vi "signal_generation_1.vi"() -> ()   [LabVIEW 2016]
uses:
  controls/State.ctl
  <vilib>/Utility/error.llb/DialogType.ctl
  <vilib>/DAQmx/write.llb/DAQmx Write (Analog Wfm 1Chan NSamp).vi
  <vilib>/DAQmx/write.llb/DAQmx Write (Analog DBL 1Chan 1Samp).vi
  <vilib>/DAQmx/read.llb/DAQmx Read (Analog 1D Wfm NChan NSamp).vi
  <vilib>/DAQmx/create/channels.llb/DAQmx Create Channel (AO-Voltage-Basic).vi
  <vilib>/DAQmx/create/channels.llb/DAQmx Create Channel (AI-Voltage-Basic).vi
  <vilib>/DAQmx/configure/timing.llb/DAQmx Timing (Sample Clock).vi
  <vilib>/DAQmx/miscellaneous.llb/DAQmx Fill In Error Info.vi
  <resource>/objmgr/daqmx.rc
  <vilib>/measure/NI_MABase.lvlib
panel:
  out "Waveform Graph 2":waveform(dbl)[](graph)=[{"t0"=timestamp(3594732894.3389087 s since 1904-01-01), "dt"=0.001, "Y"=array[1000 elements], "attributes"=variant("NI_ChannelName"=variant(string "DAQ_6363/ai0"), "NI_UnitDescription"=variant(string "Volts"))}]
  in  "DAQ channel 3 In":tag="DAQ_6363/ai0"
  out "error out":errorcluster
  in  "Number of Samples":i32=1000
  in  "Samples per Period":dbl=100.0
  in  "DAQ channel 2 In":tag="DAQ_6363/ao1"
  in  "DAQ channel 1 In":tag="DAQ_6363/ao0"
  in  "Error In (no error)":errorcluster
  in  "Exit Button":bool
  out "Status":string="Off"
  in  "TMA Voltage On/Off":bool
  out "Waveform Graph":waveform(dbl)(graph)={"t0"=timestamp(0 s since 1904-01-01), "dt"=0.001, "Y"=array[1000 elements]}
  in  "TMA Voltage":dbl=2.0 min=-10.0 max=10.0
  in  "Period (ms)":dbl=100.0 min=0.01
  in  "Amplitude (V)":dbl=2.0 min=0.0 max=30.0
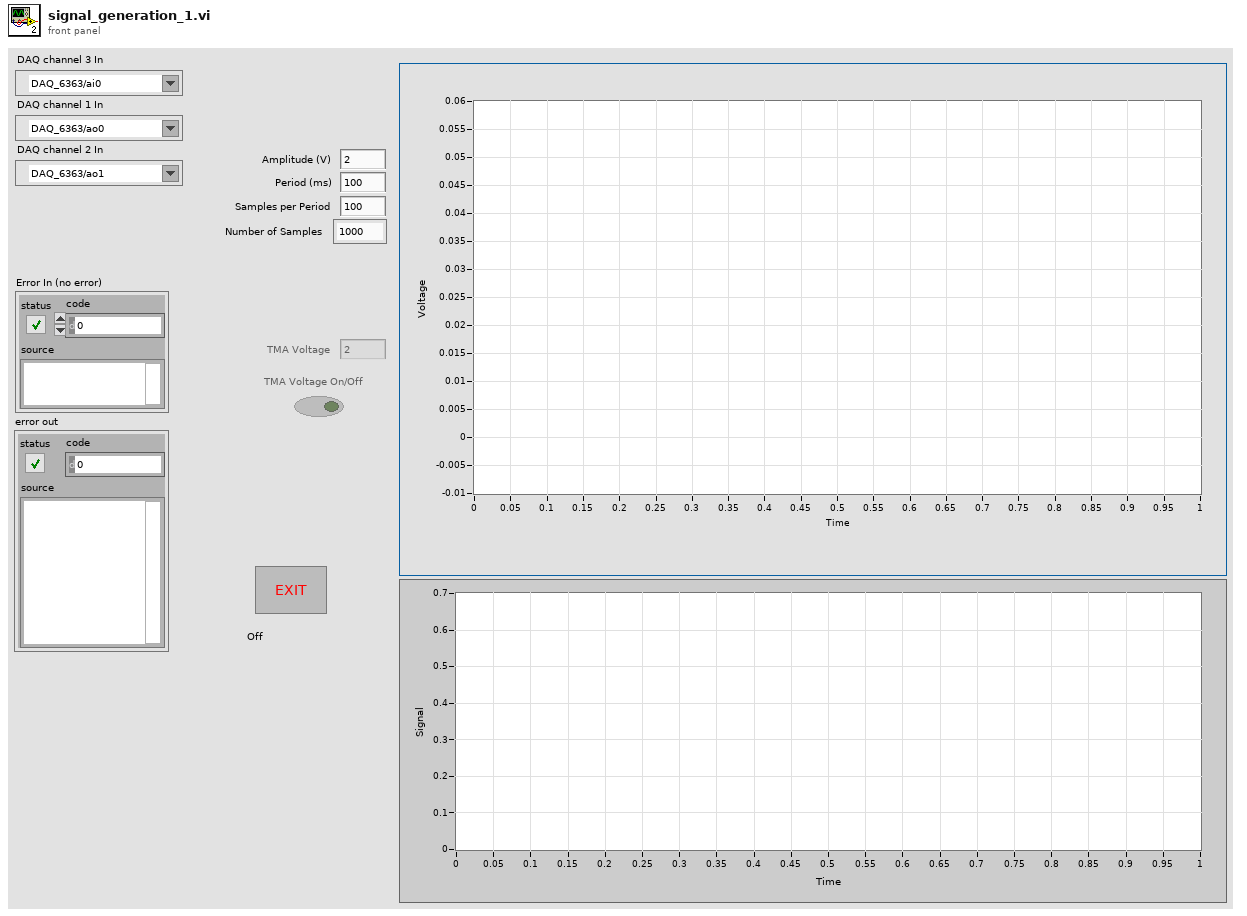
[diagram p1: front panel]
types:
  T1 = typedef "State.ctl" = enum16{"Init", "Idle", "Shutdown"}
  T2 = enum16{"Sine Wave", "Triangle Wave", "Square Wave", "Sawtooth Wave"}
  T3 = typedef "DialogType.ctl" = u16
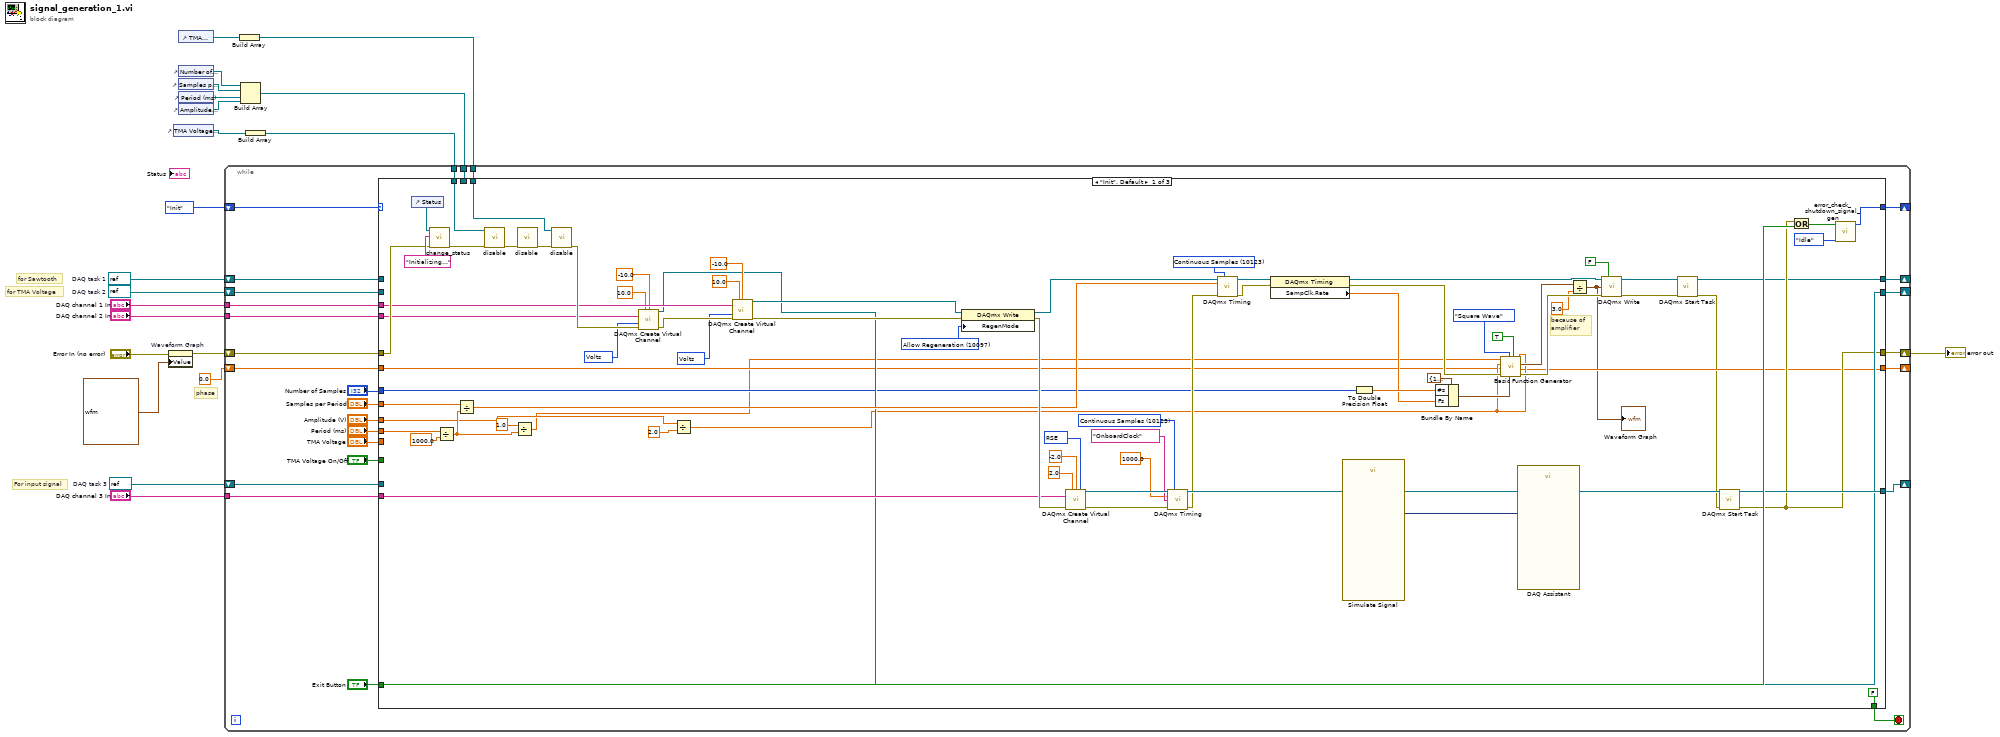
[diagram p0: block diagram]
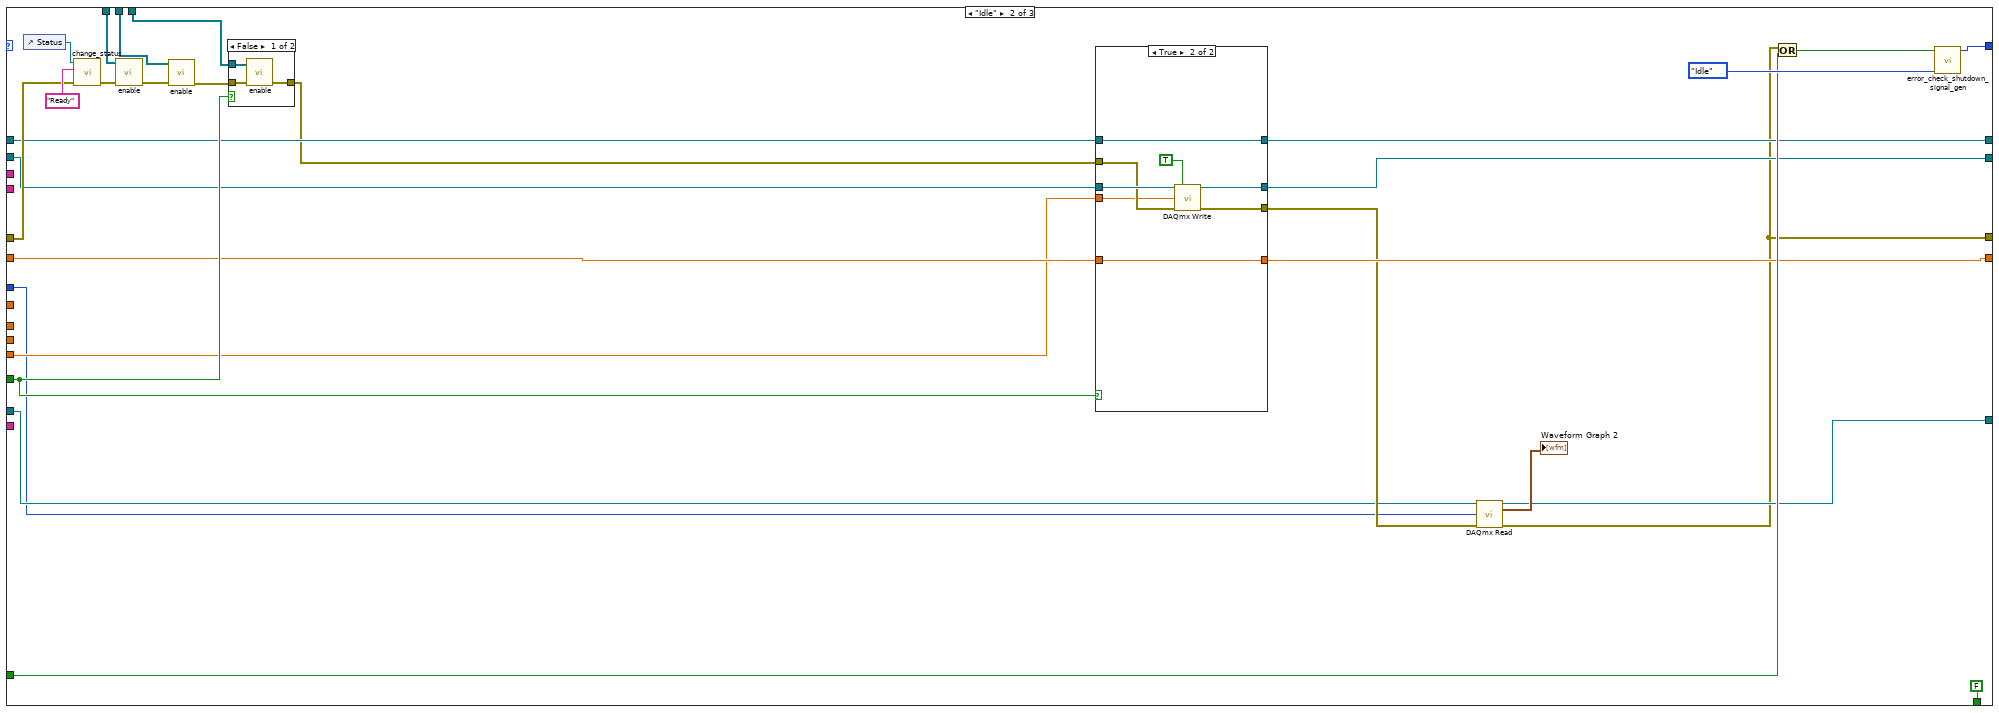
[diagram p2: hidden frame]
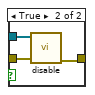
[diagram p3: hidden frame]
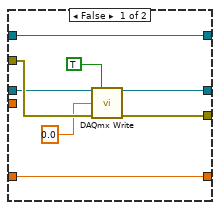
[diagram p4: hidden frame]
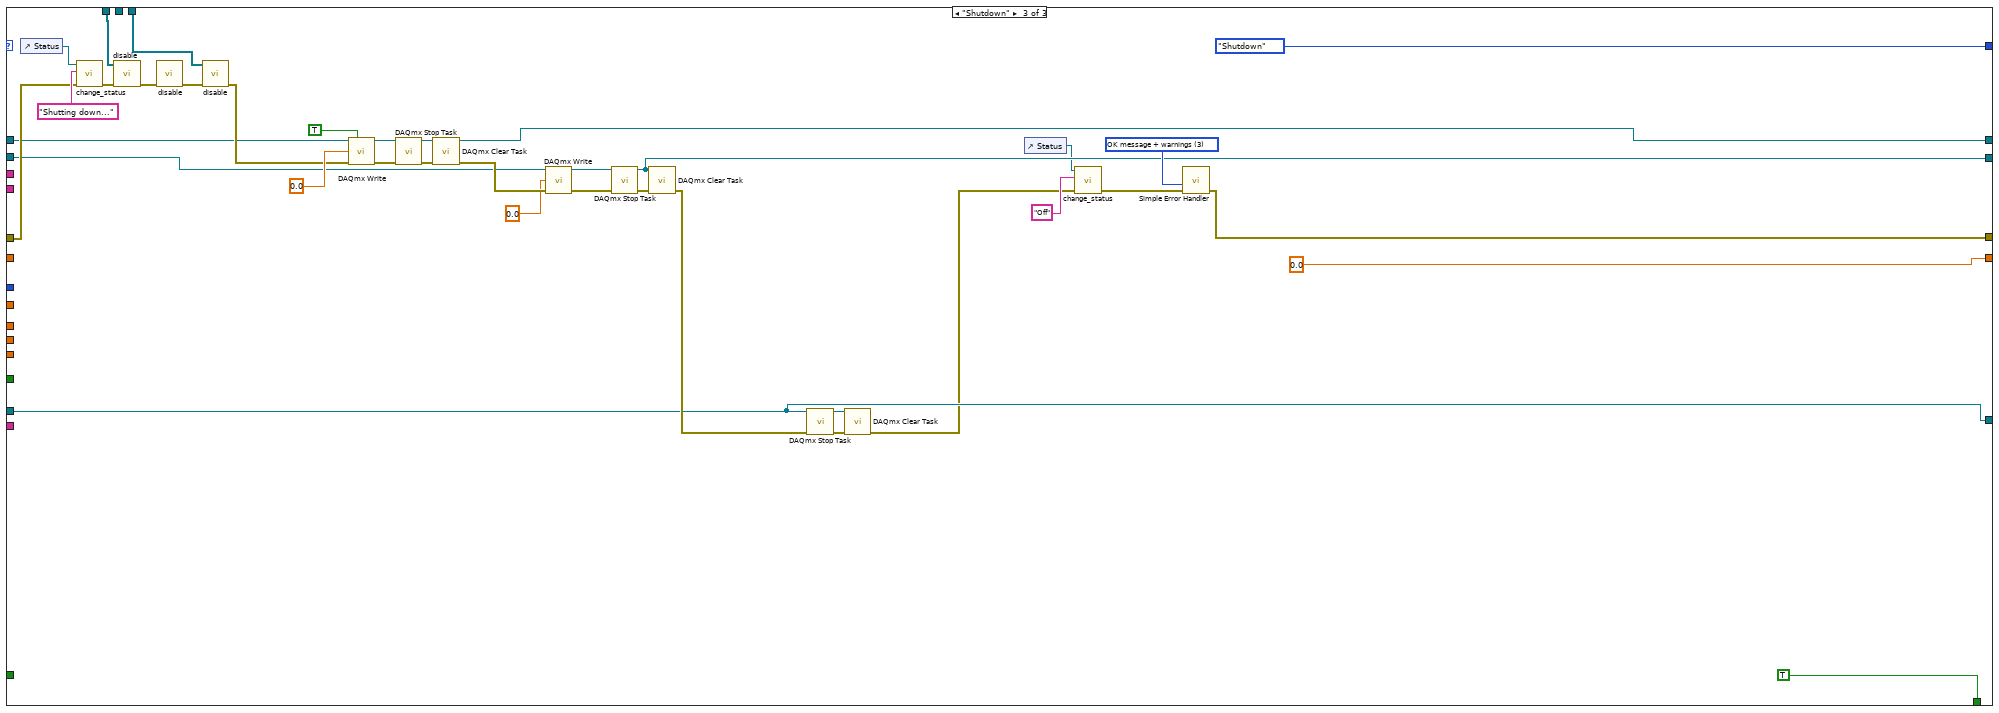
[diagram p5: hidden frame]
diagram:
  w1 = refnum<k21> refnum  # DAQ task 3
  w14 = refnum<k21> refnum  # DAQ task 1
  w13 = refnum<k21> refnum  # DAQ task 2
  # "For input signal"
  # "phase"
  # "for TMA Voltage"
  # "for Sawtooth"
  n1 = property on="Waveform Graph" class="WFGraph (strict)"(error in="Error In (no error)", "Value"=waveform(dbl) {"t0"=timestamp(0 s since 1904-01-01), "dt"=1.0, "Y"=[]} ("Waveform Graph")) -> (error out=w17:errorcluster)  [unwired: 1 in, 1 out]
  n2 = control-ref of="TMA Voltage On/Off"() -> (w20:refnum<vi>)
  n3 = control-ref of="TMA Voltage"() -> (w3:refnum<vi>)
  n4 = control-ref of="Number of Samples"() -> (w7:refnum<vi>)
  n5 = control-ref of="Samples per Period"() -> (w6:refnum<vi>)
  n6 = control-ref of="Period (ms)"() -> (w5:refnum<vi>)
  n7 = control-ref of="Amplitude (V)"() -> (w4:refnum<vi>)
  n8 = Build Array(w3) -> (w9:refnum<vi>[])
  n9 = Build Array(w7, w6, w5, w4) -> (w10:refnum<vi>[])
  n10 = Build Array(w20) -> (w19:refnum<vi>[])
  n11 = while {
    shift-right: [w34] -> _
    shift-left: State."Init" -> [w47]
    tunnel: w19 -> [w46]
    shift-right: [w33] -> w8
    shift-left: w17 -> [w41]
    tunnel: "DAQ channel 1 In" -> [w40]
    tunnel: "DAQ channel 2 In" -> [w39]
    shift-right: [w36] -> _
    shift-left: w14 -> [w38]
    shift-right: [w35] -> _
    shift-left: w13 -> [w37]
    shift-right: [w29] -> _
    shift-left: 0.0 -> [w30]
    tunnel: w10 -> [w28]
    tunnel: w9 -> [w27]
    tunnel: "DAQ channel 3 In" -> [w24]
    shift-right: [w23] -> _
    shift-left: w1 -> [w22]
    stop <- w26 stop-if-true
    n12 = case shown="\"Init\", Default" w47 {
      tunnel: w46 -> [w120 w152 w204]
      tunnel: "Amplitude (V)" -> [w73 _ _]
      tunnel: "Period (ms)" -> [w83 _ _]
      tunnel: "TMA Voltage" -> [_ w125 _]
      tunnel: "TMA Voltage On/Off" -> [_ w141 _]
      tunnel: "Exit Button" -> [w112 w145 _]
      tunnel: w41 -> [w119 w148 w207]
      tunnel: w40 -> [w116 _ _]
      tunnel: w39 -> [w117 _ _]
      tunnel: [w51 w143 w184] -> w36
      tunnel: [w78 w142 w185] -> w35
      tunnel: w38 -> [_ w130 w193]
      tunnel: w37 -> [_ w132 w188]
      tunnel: [w109 w144 State."Shutdown" ("State Out")] -> w34
      tunnel: [w77 w133 w186] -> w33
      tunnel: "Samples per Period" -> [w80 _ _]
      tunnel: "Number of Samples" -> [w70 w124 _]
      tunnel: w30 -> [w56 w131 _]
      tunnel: [w55 w138 0.0 ("phase out")] -> w29
      tunnel: w28 -> [_ w128 _]
      tunnel: w27 -> [w104 w140 w203]
      tunnel: [FALSE FALSE TRUE] -> w26
      tunnel: w24 -> [w97 _ _]
      tunnel: [w87 w134 w176] -> w23
      tunnel: w22 -> [_ w135 w176]
      frame "Init", Default {
        w86 = 10123 items=["Finite Samples"=10178, "Continuous Samples"=10123, "Hardware Timed Single Point"=12522] ("sample mode")
        w89 = 10123 items=["Finite Samples"=10178, "Continuous Samples"=10123, "Hardware Timed Single Point"=12522] ("sample mode")
        w94 = 10083 items=["Default"=-1, "RSE"=10083, "NRSE"=10078, "Differential"=10106, "Pseudodifferential"=12529] ("input terminal configuration")
        w107 = 10097 items=["Allow Regeneration"=10097, "Do Not Allow Regeneration"=10158] ("RegenMode")
        w113 = 10348 items=["Volts"=10348, "From Custom Scale"=10065] ("units")
        w114 = 10348 items=["Volts"=10348, "From Custom Scale"=10065] ("units")
        # "because of \namplifier"
        n13 = control-ref of="Status"() -> (w121:refnum<vi>)
        n14 = call "change_status.vi"("error in (no error)"=w119, "String"="Initializing...", "String in"=w121) -> ("error out"=w123:errorcluster)  [unwired: 8 in]
        n15 = Divide(x=w83, y=1000.0) -> (x/y=w75:dbl)
        n16 = Divide(x=w80, y=w75) -> (x/y=w81:dbl)
        n17 = call "disable.vi"("error in (no error)"=w123, "Array"=w120) -> ("error out"=w106:errorcluster)  [unwired: 9 in]
        n18 = Divide(x=1.0, y=w75) -> (x/y=w54:dbl)
        n19 = call "disable.vi"("error in (no error)"=w106) -> ("error out"=w105:errorcluster)  [unwired: 10 in]
        n20 = call "disable.vi"("error in (no error)"=w105, "Array"=w104) -> ("error out"=w118:errorcluster)  [unwired: 9 in]
        n21 = call-poly <vilib>:"DAQmx Create Virtual Channel.vi"("maximum value"=10.0, "minimum value"=-10.0, "physical channels"=w117, "units"=w114, "error in"=w118) -> ("task out"=w78:refnum<k21>, "error out"=w115:errorcluster)  [unwired: 9 in]
        n22 = Divide(x=w73, y=2.0) -> (x/y=w59:dbl)
        n23 = call-poly <vilib>:"DAQmx Create Virtual Channel.vi"("maximum value"=10.0, "minimum value"=-10.0, "physical channels"=w116, "units"=w113, "error in"=w115) -> ("task out"=w108:refnum<k21>, "error out"=w79:errorcluster)  [unwired: 9 in]
        n24 = property class="DAQmx Write"(reference=w108, error in=w79, "RegenMode"=w107) -> (reference out=w84:refnum<k21>, error out=w98:errorcluster)
        n25 = call-poly <vilib>:"DAQmx Create Virtual Channel.vi"("maximum value"=2.0, "minimum value"=-2.0, "input terminal configuration"=w94, "physical channels"=w97, "error in"=w98) -> ("task out"=w92:refnum<k21>, "error out"=w93:errorcluster)  [unwired: 9 in]
        n26 = call-poly <vilib>:"DAQmx Timing.vi"("task/channels in"=w92, "sample mode"=w89, "rate"=1000.0, "source"=tag "OnboardClock", "error in"=w93) -> ("task out"=w88:refnum<k21>, "error out"=w85:errorcluster)  [unwired: 9 in]
        n27 = call-poly <vilib>:"DAQmx Timing.vi"("task/channels in"=w84, "sample mode"=w86, "rate"=w81, "error in"=w85) -> ("task out"=w72:refnum<k21>, "error out"=w71:errorcluster)  [unwired: 10 in]
        n28 = property class="DAQmx Timing"(reference=w72, error in=w71) -> (reference out=w61:refnum<k21>, error out=w60:errorcluster, "SampClk.Rate"=w57:dbl)
        n29 = call "Simulate Signal"() -> ("Sawtooth"=w48:dynamicdata)  [unwired: 14 in, 1 out]
        n30 = To Double Precision Float(number=w70) -> (double precision float=w58:dbl)
        n31 = Bundle By Name(cluster=cluster{"Fs":dbl, "#s":dbl} {"Fs"=1000.0, "#s"=1000.0} ("sampling info"), "#s"=w58, "Fs"=w57) -> (w67:cluster{"Fs":dbl, "#s":dbl})
        n32 = call <vilib>:"Basic Function Generator.vi"("offset"=w59, "reset signal"=TRUE, "sampling info"=w67, "signal type"=T2."Square Wave", "error in (no error)"=w60, "phase"=w56, "amplitude"=w59, "frequency"=w54) -> ("error out"=w64:errorcluster, "phase out"=w55:dbl, "signal out"=w62:waveform(dbl))  [unwired: 1 in]
        n33 = call "DAQ Assistant"("data"=w48) -> ()  [unwired: 17 in, 2 out]
        n34 = Divide(x=w62, y=3.0) -> (x/y=w49:waveform(dbl))
        "Waveform Graph" <- w49
        n35 = call-poly <vilib>:"DAQmx Write.vi"("task/channels in"=w61, "auto start"=FALSE, "data"=w49, "error in"=w64) -> ("task out"=w52:refnum<k21>, "error out"=w53:errorcluster)  [unwired: 9 in, 1 out]
        n36 = call <vilib>:"DAQmx Start Task.vi"("task/channels in"=w52, "error in"=w53) -> ("task out"=w51:refnum<k21>, "error out"=w50:errorcluster)  [unwired: 12 in]
        n37 = call <vilib>:"DAQmx Start Task.vi"("task/channels in"=w88, "error in"=w50) -> ("task out"=w87:refnum<k21>, "error out"=w77:errorcluster)  [unwired: 12 in]
        n38 = Or(x=w77, y=w112) -> (x .or. y?=w111:bool)
        n39 = call "error_check_shutdown_signal_gen.vi"("State In"=State."Idle", "Boolean"=w111) -> ("State Out"=w109:T1)  [unwired: 9 in]
      }
      frame "Idle" {
        n40 = control-ref of="Status"() -> (w150:refnum<vi>)
        n41 = call "change_status.vi"("error in (no error)"=w148, "String"="Ready", "String in"=w150) -> ("error out"=w151:errorcluster)  [unwired: 8 in]
        n42 = call "enable.vi"("error in (no error)"=w151, "Array"=w152) -> ("error out"=w127:errorcluster)  [unwired: 9 in]
        n43 = call "enable.vi"("error in (no error)"=w127, "Array"=w128) -> ("error out"=w126:errorcluster)  [unwired: 9 in]
        n44 = case shown="False" w141 {
          tunnel: w126 -> [w155 w158]
          tunnel: [w154 w157] -> w129
          tunnel: w140 -> [w153 w156]
          frame False {
            n45 = call "enable.vi"("error in (no error)"=w155, "Array"=w153) -> ("error out"=w154:errorcluster)  [unwired: 9 in]
          }
          frame True {
            n46 = call "disable.vi"("error in (no error)"=w158, "Array"=w156) -> ("error out"=w157:errorcluster)  [unwired: 9 in]
          }
        }
        n47 = case shown="True" w141 {
          tunnel: w130 -> [w166 w174]
          tunnel: w129 -> [w164 w171]
          tunnel: w132 -> [w163 w173]
          tunnel: [w166 w174] -> w143
          tunnel: [w162 w172] -> w142
          tunnel: [w165 w170] -> w136
          tunnel: w131 -> [w159 w168]
          tunnel: [w159 w168] -> w138
          tunnel: w125 -> [_ w167]
          frame False {
            n48 = call-poly <vilib>:"DAQmx Write.vi"("task/channels in"=w163, "auto start"=TRUE, "data"=0.0, "error in"=w164) -> ("task out"=w162:refnum<k21>, "error out"=w165:errorcluster)  [unwired: 9 in, 1 out]
          }
          frame True {
            n49 = call-poly <vilib>:"DAQmx Write.vi"("task/channels in"=w173, "auto start"=TRUE, "data"=w167, "error in"=w171) -> ("task out"=w172:refnum<k21>, "error out"=w170:errorcluster)  [unwired: 9 in, 1 out]
          }
        }
        n50 = call-poly <vilib>:"DAQmx Read.vi"("task/channels in"=w135, "number of samples per channel"=w124, "error in"=w136) -> ("task out"=w134:refnum<k21>, "data"=→"Waveform Graph 2":waveform(dbl)[], "error out"=w133:errorcluster)  [unwired: 10 in]
        n51 = Or(x=w133, y=w145) -> (x .or. y?=w147:bool)
        n52 = call "error_check_shutdown_signal_gen.vi"("State In"=State."Idle", "Boolean"=w147) -> ("State Out"=w144:T1)  [unwired: 9 in]
      }
      frame "Shutdown" {
        w199 = T3 3 items=["no dialog", "OK message", "continue or stop message", "OK message + warnings", "continue/stop + warnings"] ("type of dialog (OK msg:1)")
        n53 = control-ref of="Status"() -> (w210:refnum<vi>)
        n54 = call "change_status.vi"("error in (no error)"=w207, "String"="Shutting down...", "String in"=w210) -> ("error out"=w208:errorcluster)  [unwired: 8 in]
        n55 = call "disable.vi"("error in (no error)"=w208, "Array"=w204) -> ("error out"=w206:errorcluster)  [unwired: 9 in]
        n56 = call "disable.vi"("error in (no error)"=w206) -> ("error out"=w205:errorcluster)  [unwired: 10 in]
        n57 = call "disable.vi"("error in (no error)"=w205, "Array"=w203) -> ("error out"=w194:errorcluster)  [unwired: 9 in]
        n58 = call-poly <vilib>:"DAQmx Write.vi"("task/channels in"=w193, "auto start"=TRUE, "data"=0.0, "error in"=w194) -> ("task out"=w195:refnum<k21>, "error out"=w196:errorcluster)  [unwired: 9 in, 1 out]
        n59 = call <vilib>:"DAQmx Stop Task.vi"("task/channels in"=w195, "error in"=w196) -> ("task out"=w184:refnum<k21>, "error out"=w200:errorcluster)  [unwired: 12 in]
        n60 = call <vilib>:"DAQmx Clear Task.vi"("task in"=w184, "error in"=w200) -> ("error out"=w192:errorcluster)  [unwired: 13 in]
        n61 = call-poly <vilib>:"DAQmx Write.vi"("task/channels in"=w188, "data"=0.0, "error in"=w192) -> ("task out"=w190:refnum<k21>, "error out"=w191:errorcluster)  [unwired: 10 in, 1 out]
        n62 = call <vilib>:"DAQmx Stop Task.vi"("task/channels in"=w190, "error in"=w191) -> ("task out"=w185:refnum<k21>, "error out"=w198:errorcluster)  [unwired: 12 in]
        n63 = call <vilib>:"DAQmx Clear Task.vi"("task in"=w185, "error in"=w198) -> ("error out"=w177:errorcluster)  [unwired: 13 in]
        n64 = call <vilib>:"DAQmx Stop Task.vi"("task/channels in"=w176, "error in"=w177) -> ("task out"=w178:refnum<k21>, "error out"=w179:errorcluster)  [unwired: 12 in]
        n65 = call <vilib>:"DAQmx Clear Task.vi"("task in"=w178, "error in"=w179) -> ("error out"=w175:errorcluster)  [unwired: 13 in]
        n66 = control-ref of="Status"() -> (w181:refnum<vi>)
        n67 = call "change_status.vi"("error in (no error)"=w175, "String"="Off", "String in"=w181) -> ("error out"=w182:errorcluster)  [unwired: 8 in]
        n68 = call <vilib>:"Simple Error Handler.vi"("type of dialog (OK msg:1)"=w199, "error in (no error)"=w182) -> ("error out"=w186:errorcluster)  [unwired: 3 in, 4 out]
      }
    }
  }
  "error out" <- w8
